vi "Extract Parameters(private).vi"(8 "error in":errorcluster, 11 "Analyze objs":refnum<class "Analyze BaseClass.lvclass">[](array[class])) -> (0 "error out":errorcluster, 3 "Parameters":refnum<class "Analyze Parameter Base.lvclass">[](array[class]))   [LabVIEW 2014, in "Analyze Actor.lvlib" / "Analyze Actor.lvclass"]
uses:
  Analyze Actor.lvclass
  Analyze Classes/Analyze BaseClass/Analyze BaseClass/Analyze BaseClass.lvclass
  Analyze Parameter/Analyze Parameter Base/Analyze Parameter Base.lvclass
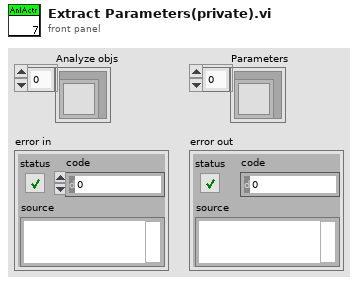
[diagram p1: front panel]
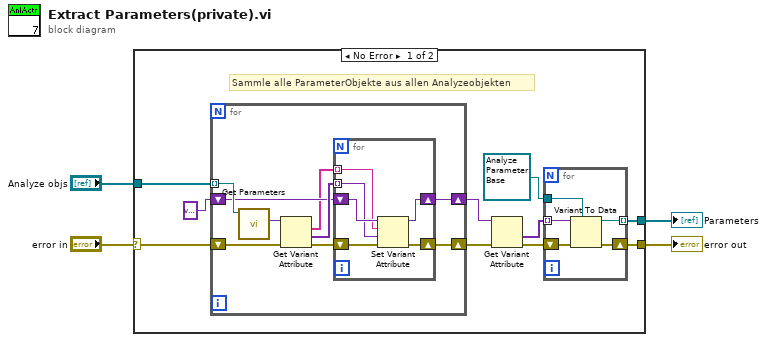
[diagram p0: block diagram]
diagram:
  n1 = case shown="No Error" "error in" {
    selector: "error in" -> [w5 w35]
    tunnel: "Analyze objs" -> [w14 _]
    tunnel: [w7 _] -> w3
    tunnel: [w6 w35] -> w2
    frame No Error {
      # "Sammle alle ParameterObjekte aus allen Analyzeobjekten"
      n2 = for {
        tunnel: w14 -> [w28] mode=indexing
        shift-right: [w24] -> w9
        shift-left: variant ("Variant") -> [w25]
        shift-right: [w21] -> w8
        shift-left: w5 -> [w20]
        n3 = call-dynamic "Get Parameters.vi"("Analyze BaseClass in"=w28) -> ("Parameters out"=w27:variant)  [unwired: 8 in, 2 out]
        n4 = Get Variant Attribute(Variant=w27, error in=w20) -> (names=w23:string[], values=w26:variant[], error out=w22:errorcluster)  [unwired: 2 in, 1 out]
        n5 = for {
          tunnel: w26 -> [w31] mode=indexing
          shift-right: [w33] -> w24
          shift-left: w25 -> [w34]
          tunnel: w23 -> [w32] mode=indexing
          shift-right: [w29] -> w21
          shift-left: w22 -> [w30]
          n6 = Set Variant Attribute(Variant=w34, name=w32, value=w31, error in=w30) -> (Variant out=w33:variant, error out=w29:errorcluster)  [unwired: 1 out]
        }
      }
      n7 = Get Variant Attribute(Variant=w9, error in=w8) -> (values=w11:variant[], error out=w12:errorcluster)  [unwired: 2 in, 2 out]
      n8 = for {
        tunnel: w11 -> [w18] mode=indexing
        tunnel: refnum<class "Analyze Parameter Base.lvclass"> refnum ("Analyze Parameter Base.lvclass") -> [w19]
        tunnel: [w16] -> w7 mode=indexing
        shift-right: [w15] -> w6
        shift-left: w12 -> [w17]
        n9 = Variant To Data(error in=w17, type=w19, Variant=w18) -> (data=w16:refnum<class "Analyze Parameter Base.lvclass">, error out=w15:errorcluster)
      }
    }
    frame Error {
    }
  }
  "Parameters" <- w3
  "error out" <- w2
